vi "Process.vi"(8 "error in (no error)":errorcluster, 10 "Pound in":refnum<class "Pound.lvclass">, 11 "Qbus in":refnum<class "Qbus.lvclass">) -> (0 "error out":errorcluster)   [LabVIEW 2017, in "McsaAnalysisLowRate.lvlib"]
doc: "Calculates features and spectral bands, or trends, from waveforms that the channels in a data group acquire. Subsequent processes can evaluate this feature data to trigger alarms, collect data sets, and perform other operations."
uses:
  <vilib>/addons/InsightCM/Devices/Shared/Mcsa/McsaAnalysisLowRate/McsaAnalysisLowRate.lvlib
  <vilib>/addons/Qbus/Qbus.lvclass
  <vilib>/NI/Software Watchdog/Pound/Pound.lvclass
  <vilib>/addons/InsightCM/Devices/Shared/Mcsa/McsaAnalysisLowRate/controls/Config.ctl
  <vilib>/addons/InsightCM/Devices/Shared/Mcsa/McsaAnalysisLowRate/controls/Group.ctl
  <vilib>/addons/InsightCM/Utilities/Analysis/MCSA/controls/McsaChannel.ctl
  <vilib>/addons/InsightCM/Utilities/Analysis/Shared/controls/Feature.ctl
  <vilib>/addons/InsightCM/Utilities/Analysis/Shared/controls/AmplitudeScale.ctl
  <vilib>/addons/InsightCM/MessageBus/Base/controls/KeyValuePair.ctl
  <vilib>/addons/InsightCM/Utilities/Analysis/MCSA/controls/McsaChannelPhasor.ctl
  <vilib>/addons/InsightCM/Utilities/Analysis/MCSA/controls/McsaMotor.ctl
  <vilib>/addons/InsightCM/Utilities/Analysis/MCSA/controls/MotorCalculationCache.ctl
  <vilib>/addons/Electrical Power/Basic/Measurement/subVIs/basic_Power Value.ctl
  <vilib>/addons/InsightCM/Utilities/Analysis/MCSA/controls/TorqueLoadEfficiency.ctl
  <vilib>/addons/InsightCM/Utilities/Analysis/MCSA/controls/WorkingCurrent.ctl
  <vilib>/NI/Software Watchdog/Watchdog/Watchdog.lvclass
  <vilib>/addons/InsightCM/Devices/Shared/Common/DataFlow/DataFlow.lvlib
  <vilib>/addons/InsightCM/Utilities/Analysis/Shared/AnalysisHelper.lvlib
  <vilib>/addons/InsightCM/Utilities/GlobalConfiguration/GlobalConfiguration.lvlib
  <vilib>/addons/InsightCM/Devices/Shared/Common/DataEventCreator/DataEventCreator.lvlib
  <vilib>/addons/InsightCM/Utilities/Analysis/MCSA/McsaAnalysisFunctions.lvlib
  <vilib>/addons/TraceLogger/TraceLogger.lvlib
  <vilib>/addons/InsightCM/Devices/Shared/Mcsa/McsaDataEventCreator/McsaDataEventCreator.lvlib
  <vilib>/addons/InsightCM/Devices/Shared/Mcsa/McsaResourceSchedulerLR/McsaResourceSchedulerLR.lvlib
  <vilib>/addons/Electrical Power/Basic/NI_EP_Basic.lvlib
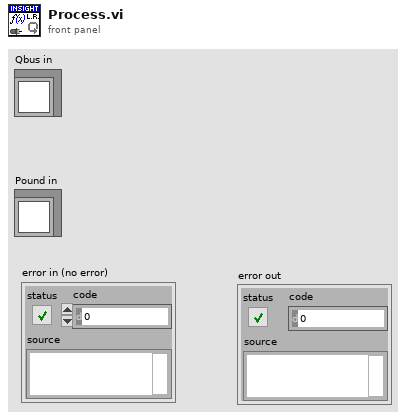
[diagram p1: front panel]
types:
  T1 = typedef "McsaAnalysisLowRate.lvlib/Config.ctl" = cluster{"Device Name":string, "Groups":T2[], "Working Current":T12, "Max Group":i32}
  T2 = typedef "McsaAnalysisLowRate.lvlib/Group.ctl" = cluster{"Name":string, "Channels":T3[], "Channel Phasors":T7[], "Motor Info":T8, "Calculation Cache":T9}
  T3 = typedef "McsaAnalysisFunctions.lvlib/McsaChannel.ctl" = cluster{"Name":string, "Id":string, "Type":string, "Wiring Configuration":string, "Nominal Line Voltage":dbl, "Phase A Channel":string, "Phase B Channel":string, "Phase C Channel":string, "Channel Status":string, "Features":T4[], "Data Valid":bool, "Acq Timestamp":timestamp, "Channel Properties":T6[], "Torque Waveform Unit":string}
  T4 = typedef "AnalysisHelper.lvlib/Feature.ctl" = cluster{"MetricType":string, "TdmsPropName":string, "DisplayName":string, "Unit":string, "Use Volts":bool, "Value":dbl, "Tag Id":string, "Properties":variant, "Amplitude Scale":T5, "valid":bool}
  T5 = typedef "AnalysisHelper.lvlib/AmplitudeScale.ctl" = enum16{"rms", "peak", "pk-pk"}
  T6 = typedef "KeyValuePair.ctl" = cluster{"Key":string, "Value":string}
  T7 = typedef "McsaAnalysisFunctions.lvlib/McsaChannelPhasor.ctl" = cluster{"channel name":string, "Magnitude":dbl, "Phase":dbl, "Frequency":dbl, "phasor":cdb, "Phase Order (A/B/C)":string}
  T8 = typedef "McsaAnalysisFunctions.lvlib/McsaMotor.ctl" = cluster{"Model":string, "Manufacturer":string, "Serial Number":string, "Horsepower":dbl, "Horsepower Unit":string, "Full Load Speed":dbl, "Synchronous Speed":dbl, "Rated Volts":dbl, "Full Load Amps":dbl, "Frequency":dbl, "Service Factor":dbl, "Efficiency":dbl, "Efficiency @ 75% Load":dbl, "Efficiency @ 50% Load":dbl, "Efficiency @ 25% Load":dbl, "Power Factor":dbl, "VoltageBus":string, "VoltageBus ID":string, "Stator Resistance":dbl, "Estimate Stator Resistance":bool}
  T9 = typedef "McsaAnalysisFunctions.lvlib/MotorCalculationCache.ctl" = cluster{"Power Init":bool, "power value":T10, "Pout Init":bool, "Pout":T11, "Derating Factor Init":bool, "derating factor":sgl, "torque waveform":waveform(dbl), "invalid estimation":bool}
  T10 = typedef "NI_EP_Basic.lvlib/basic_Power Value.ctl" = cluster{"active power [W]":dbl, "apparent power [VA]":dbl, "reactive power [VAR]":dbl, "power factor":dbl}
  T11 = typedef "McsaAnalysisFunctions.lvlib/TorqueLoadEfficiency.ctl" = cluster{"torque [Nm]":dbl, "load [kW]":dbl, "efficiency [%]":dbl, "percent load [%]":dbl}
  T12 = typedef "McsaAnalysisFunctions.lvlib/WorkingCurrent.ctl" = cluster{"Min Current (%FLA)":dbl, "Max Current (%FLA)":dbl}
  T13 = typedef "DataEventCreator.lvlib/RegisterTrendPoints.ctl" = cluster{"DataGroup":string, "Trends":T14[]}
  T14 = typedef "DataEventCreator.lvlib/Registry_Trend.ctl" = cluster{"TrendPointId":string, "DataSetName":string, "HighRate":bool, "Always Send":bool}
  T15 = typedef "DataFlow.lvlib/Data.ctl" = cluster{"DataGroup":string, "Waveforms":T16, "Map":T17, "Type":T18}
  T16 = typedef "wfmSGL_DVR.ctl" = refnum<data-value>
  T17 = typedef "PointValueMap.lvlib/PointMap.ctl" = refnum<data-value>
  T18 = typedef "DataFlow.lvlib/Type.ctl" = enum16{"High Rate", "Low Rate", "Burst Mode"}
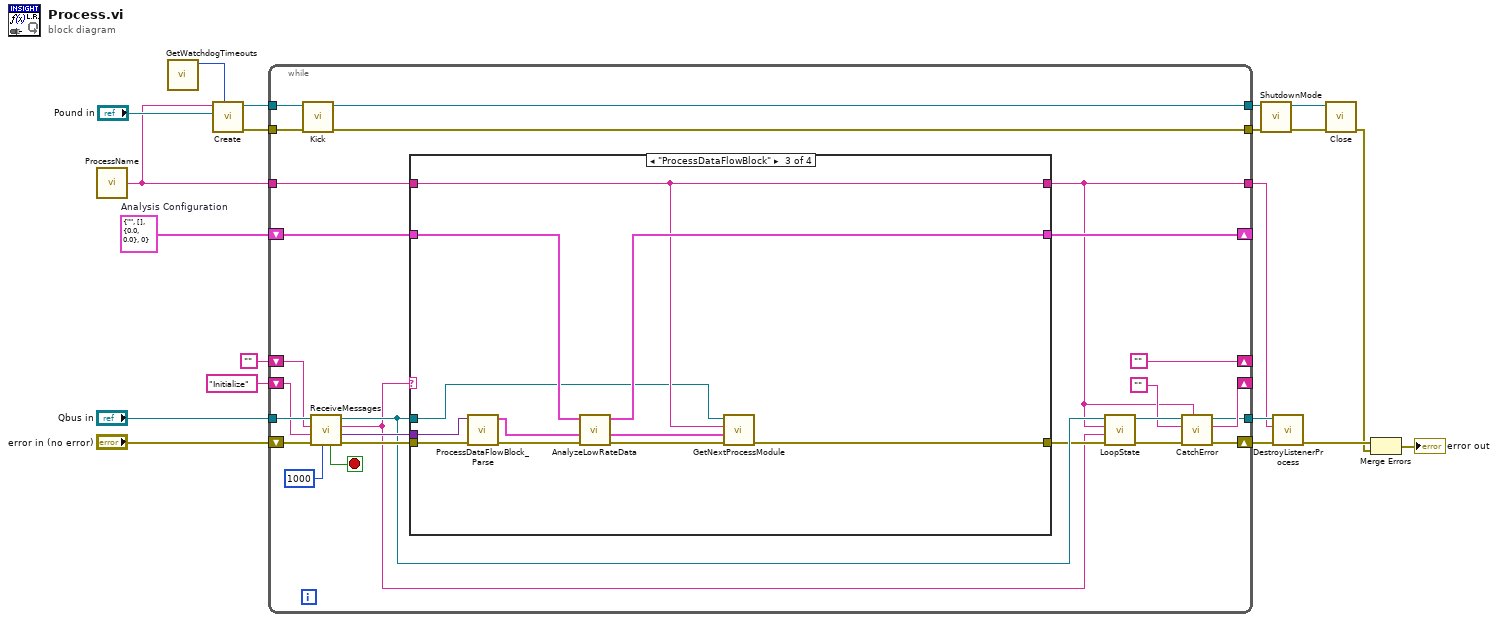
[diagram p0: block diagram]
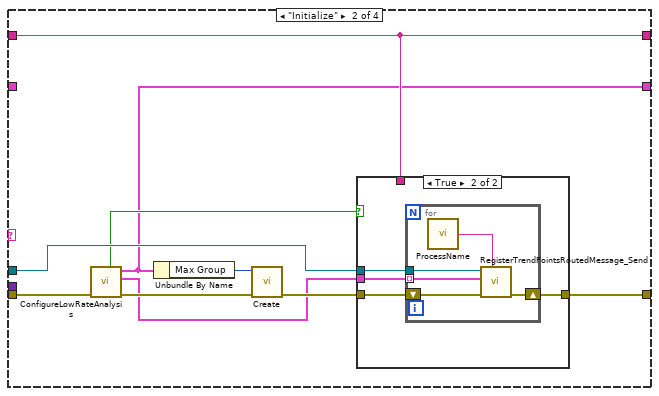
[diagram p3: hidden frame]
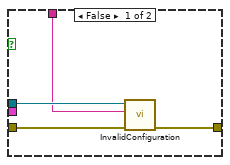
[diagram p4: hidden frame]
diagram:
  w1 = T1 {"Device Name"="", "Groups"=[], "Working Current"={"Min Current (%FLA)"=0.0, "Max Current (%FLA)"=0.0}, "Max Group"=0}  # Analysis Configuration
  n1 = call <vilib>:"ProcessName.vi"() -> ("ProcessName"=w2:string)  [unwired: 5 in]
  n2 = call <vilib>:"GetWatchdogTimeouts.vi"() -> ("software timeout"=w3:u32)  [unwired: 10 in, 1 out]
  n3 = call <vilib>:"Create.vi"("Execution Timeout (ms)"=w3, "Pound"="Pound in", "Name"=w2) -> ("error out"=w10:errorcluster, "Watchdog"=w11:refnum<data-value>)  [unwired: 7 in]
  n4 = while {
    shift-right: [""] -> _
    shift-left: "" -> [w40]
    shift-right: [w46] -> _
    shift-left: w1 -> [w45]
    shift-right: [w27] -> _
    shift-left: "Initialize" ("MsgName") -> [w38]
    tunnel: w2 -> [w33]
    tunnel: [w26] -> w16
    tunnel: [w24] -> w15
    tunnel: "Qbus in" -> [w43]
    tunnel: [w37] -> w13
    tunnel: [w36] -> w12
    tunnel: w11 -> [w35]
    tunnel: w10 -> [w34]
    shift-right: [w25] -> w17
    shift-left: "error in (no error)" -> [w39]
    stop <- w22 stop-if-true
    n5 = call <vilib>:"Kick.vi"("error in (no error)"=w34, "Watchdog"=w35) -> ("error out"=w37:errorcluster, "Watchdog"=w36:refnum<data-value>)  [unwired: 8 in]
    n6 = call <vilib>:"ReceiveMessages.vi"("Timeout(100)"=1000, "error in (no error)"=w39, "Priority Action"=w38, "Default Action"=w40, "Qbus in"=w43) -> ("error out"=w41:errorcluster, "MsgValue"=w42:variant, "Action"=w23:string, "Qbus out"=w32:refnum<class "Qbus.lvclass">, "Exit"=w22:bool)  [unwired: 2 in]
    n7 = case shown="\"ProcessDataFlowBlock\"" w23 {
      tunnel: w41 -> [w49 w51 w81 w85]
      tunnel: [w49 w58 w76 w85] -> w31
      tunnel: w42 -> [_ _ w80 _]
      tunnel: [w48 w54 w82 w84] -> w46
      tunnel: w45 -> [w48 _ w83 w84]
      tunnel: w32 -> [_ w59 w75 _]
      tunnel: [w47 w56 w77 w86] -> w24
      tunnel: w33 -> [w47 w56 w77 w86]
      frame Default {
      }
      frame "Initialize" {
        n8 = call <vilib>:"ConfigureLowRateAnalysis.vi"("error in (no error)"=w51) -> ("error out"=w53:errorcluster, "register trends"=w50:T13[], "analysis config"=w54:T1, "all config found?"=w57:bool)  [unwired: 7 in]
        n9 = Unbundle By Name(w54) -> ("Max Group"=w52:i32)
        n10 = call <vilib>:"Create.vi"("error in (no error)"=w53, "count"=w52) -> ("error out"=w55:errorcluster)  [unwired: 9 in]
        n11 = case shown="True" w57 {
          tunnel: w59 -> [w63 w67]
          tunnel: w50 -> [_ w66]
          tunnel: w55 -> [w62 w65]
          tunnel: [w61 w64] -> w58
          tunnel: w56 -> [w60 _]
          frame False {
            n12 = call <vilib>:"InvalidConfiguration.vi"("error in (no error)"=w62, "description"=w60, "Qbus in"=w63) -> ("error out"=w61:errorcluster)  [unwired: 7 in, 1 out]
          }
          frame True {
            n13 = for {
              tunnel: w66 -> [w72] mode=indexing
              shift-right: [w70] -> w64
              shift-left: w65 -> [w71]
              tunnel: w67 -> [w69]
              n14 = call <vilib>:"ProcessName.vi"() -> ("process name"=w68:string)  [unwired: 5 in]
              n15 = call <vilib>:"RegisterTrendPointsRoutedMessage_Send.vi"("data event creator process name"=w68, "error in (no error)"=w71, "register trend"=w72, "Qbus in"=w69) -> ("error out"=w70:errorcluster)  [unwired: 6 in, 1 out]
            }
          }
        }
      }
      frame "ProcessDataFlowBlock" {
        n16 = call <vilib>:"ProcessDataFlowBlock_Parse.vi"("error in (no error)"=w81, "body"=w80) -> ("error out"=w74:errorcluster, "data"=w78:T15)  [unwired: 8 in]
        n17 = call <vilib>:"AnalyzeLowRateData.vi"("error in (no error)"=w74, "data in"=w78, "Analysis Configuration In"=w83) -> ("error out"=w73:errorcluster, "data out"=w79:T15, "Analysis Configuration Out"=w82:T1)  [unwired: 6 in]
        n18 = call <vilib>:"GetNextProcessModule.vi"("error in (no error)"=w73, "data"=w79, "source"=w77, "Qbus in"=w75) -> ("error out"=w76:errorcluster)  [unwired: 6 in, 1 out]
      }
      frame "Exit" {
      }
    }
    n19 = call <vilib>:"LoopState.vi"("error in (no error)"=w31, "loop action"=w23, "process name"=w24, "Qbus in"=w32) -> ("error out"=w28:errorcluster, "Qbus out"=w30:refnum<class "Qbus.lvclass">)  [unwired: 6 in]
    n20 = call <vilib>:"CatchError.vi"("source"=w24, "error in (no error)"=w28, "next action in"="", "Qbus in"=w30) -> ("error out"=w25:errorcluster, "next action out"=w27:string, "Qbus out"=w26:refnum<class "Qbus.lvclass">)  [unwired: 5 in]
  }
  n21 = call <vilib>:"ShutdownMode.vi"("error in (no error)"=w13, "Watchdog"=w12) -> ("error out"=w18:errorcluster, "Watchdog"=w19:refnum<data-value>)  [unwired: 8 in]
  n22 = call <vilib>:"DestroyListenerProcess.vi"("error in (no error)"=w17, "process name"=w15, "Qbus in"=w16) -> ("error in (no error)"=w9:errorcluster)  [unwired: 7 in, 1 out]
  n23 = call <vilib>:"Close.vi"("error in (no error)"=w18, "Watchdog"=w19) -> ("error out"=w8:errorcluster)  [unwired: 9 in]
  n24 = Merge Errors(w9, w8) -> (→"error out":errorcluster)
